vi "Initialize.vi"(8 "error in":errorcluster, 10 "parameters":variant, 11 "current in":refnum<class "current node.lvclass">) -> (0 "error out":errorcluster, 2 "summary":T2[](array[typedef]), 3 "data value reference":T1)   [LabVIEW 2014, in "current node.lvclass"]
doc: "This Vi initializes the data of a node its default state.\nThe object is not created inside of this ViI, beacuase it is created from a File depending on user selection."
uses:
  current node.lvclass
  <vilib>/NI/Configuration Framework/Node/Summary.ctl
  <vilib>/NI/Configuration Framework/Node/NodeRef.ctl
  <vilib>/NI/Configuration Framework/Node/NISE_CEF_Node.lvclass
  channel configuration/ChannelData.ctl
  channel node/Write Channel info.vi
  channel node/channel node.lvclass
  channel configuration/channel configuration.lvclass
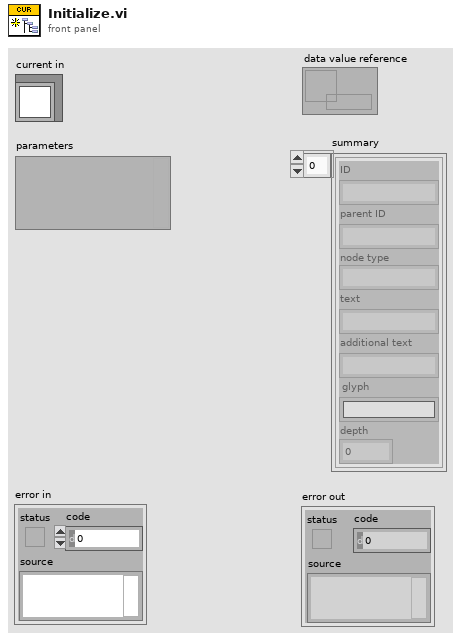
[diagram p1: front panel]
types:
  T1 = typedef "NISE_CEF_Node.lvclass/NodeRef.ctl" = refnum<data-value>
  T2 = typedef "NISE_CEF_Node.lvclass/Summary.ctl" = cluster{"ID":string, "parent ID":string, "node type":string, "text":string, "additional text":string, "glyph":string, "depth":i32}
  T3 = typedef "channel configuration.lvclass/ChannelData.ctl" = cluster{"channel group":string, "channel name":string, "IO":string, "sensor ID":string, "description":string, "system":string, "channel type":string}
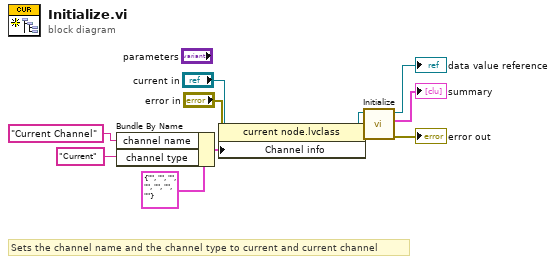
[diagram p0: block diagram]
diagram:
  # "Sets the channel name and the channel type to current and current channel"
  n1 = Bundle By Name(cluster=T3 {"channel group"="", "channel name"="", "IO"="", "sensor ID"="", "description"="", "system"="", "channel type"=""} ("channel info"), "channel name"="Current Channel" ("channel Name"), "channel type"="Current" ("channelType")) -> (w7:T3)
  n2 = property class="current node.lvclass"(reference="current in", error in="error in", "Channel info"=w7) -> (reference out=w4:refnum<class "current node.lvclass">, error out=w5:errorcluster)
  n3 = call-parent "Initialize.vi"("error in"=w5, "node in"=w4) -> ("error out"=→"error out":errorcluster, "summary"=→"summary":T2[], "data value reference"=→"data value reference":T1)  [unwired: 7 in]
